vi "Status to color.vi"(11 "Byte":u8) -> (3 "Numeric":u32)   [LabVIEW 2016]
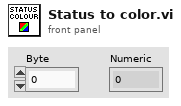
[diagram p1: front panel]
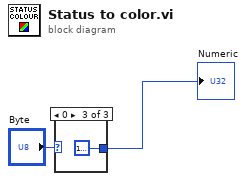
[diagram p0: block diagram]
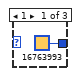
[diagram p2: hidden frame]
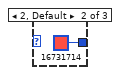
[diagram p3: hidden frame]
diagram:
  n1 = case shown="0" "Byte" {
    tunnel: [u32 16763993 u32 16731714 u32 16777238] -> w2
    frame 1 {
    }
    frame 2, Default {
    }
    frame 0 {
    }
  }
  "Numeric" <- w2
